vi "Update DVR Constant.vi"() -> ()   [LabVIEW 2020]
uses:
  <vilib>/Utility/traverseref.llb/TRef TravTarget.ctl
  <vilib>/Utility/traverseref.llb/VI Scripting - Traverse.lvlib
panel:
  out "Typedef:Path":path
  out "Class Name":string
  out "VI Name":string
  out "Basic Object Flags":u32
  out "Label.Text":string
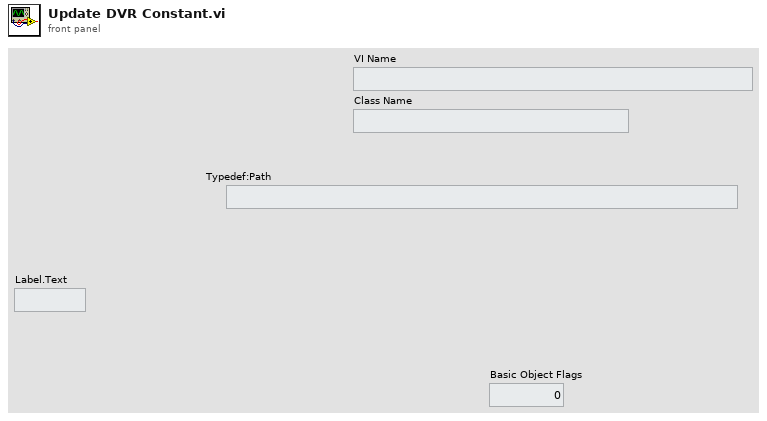
[diagram p1: front panel]
types:
  T1 = typedef "TRef TravTarget.ctl" = enum16{"FP", "BD", "Other"}
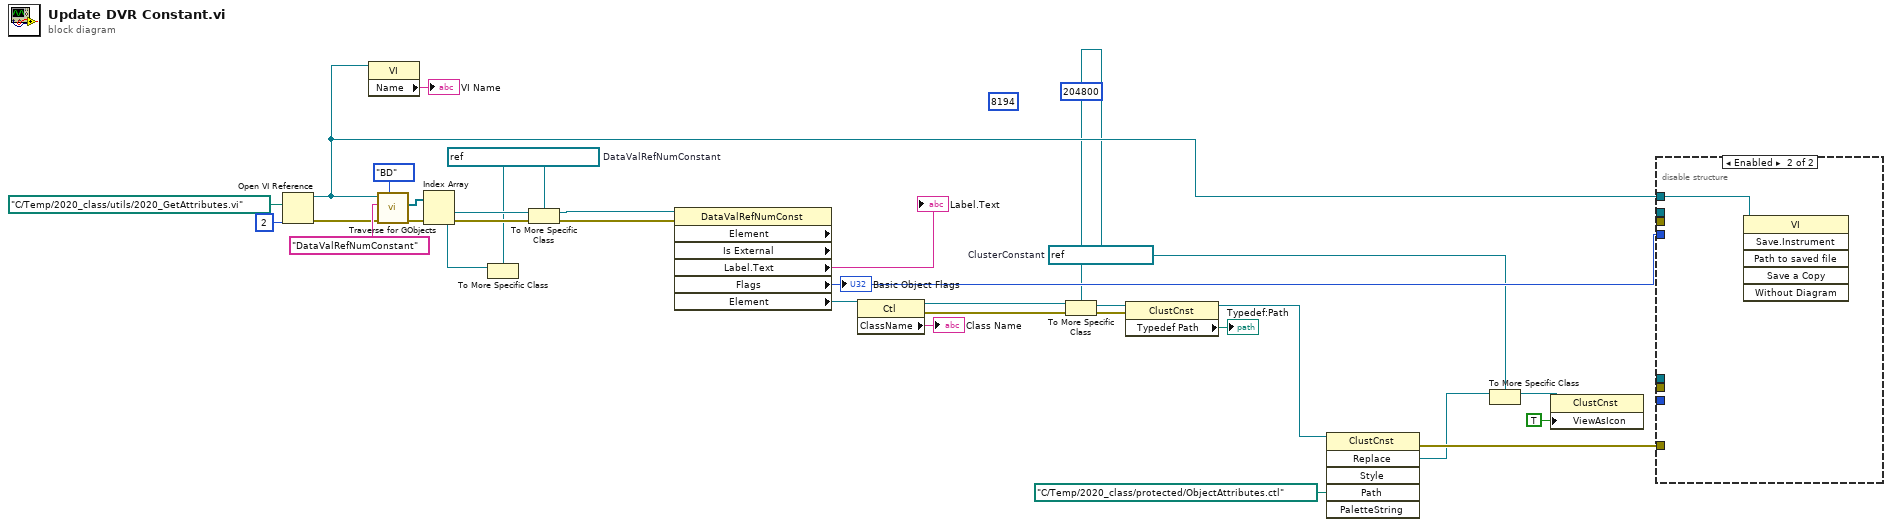
[diagram p0: block diagram]
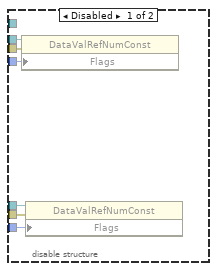
[diagram p2: hidden frame]
diagram:
  w3 = refnum<vi> refnum  # ClusterConstant
  (unwired) u32 204800 ("Basic Object Flags")
  (unwired) u32 8194 ("Basic Object Flags 2")
  w20 = refnum<vi> refnum  # DataValRefNumConstant
  n1 = Open VI Reference(vi path=path "C:/Temp/2020_class/utils/2020_GetAttributes.vi", options=2) -> (vi reference=w15:refnum<vi>, error out=w16:errorcluster)  [unwired: 4 in]
  n2 = property class="VI"(reference=w15) -> ("Name"=→"VI Name":string)  [unwired: 1 in, 2 out]
  n3 = call <vilib>:"Traverse for GObjects.vi"("Traverse Target"=TRef_TravTarget."BD", "error in (no error)"=w16, "Class Name"="DataValRefNumConstant", "VI Refnum"=w15) -> ("error out"=w25:errorcluster, "References"=w27:refnum<vi>[])  [unwired: 4 in, 2 out]
  n4 = Index Array(array=w27) -> (element #1=w26:refnum<vi>, element #2=w21:refnum<vi>)  [unwired: 2 in]
  n5 = To More Specific Class(target class=w20, reference=w21) -> ()  [unwired: 1 in, 2 out]
  n6 = To More Specific Class(target class=w20, reference=w26, error in=w25) -> (specific class reference=w22:refnum<vi>, error out=w24:errorcluster)
  n7 = property class="DataValRefNumConst" props=["Element", "Is External", "Label", "Text", "Flags", "Element"](reference=w22, error in=w24) -> ("Label.Text"=→"Label.Text":string, "Flags"=w19:u32, "Element"=w14:refnum<vi>)  [unwired: 4 out]
  "Basic Object Flags" <- w19
  n8 = property class="Ctl"(reference=w14) -> (reference out=w12:refnum<vi>, error out=w11:errorcluster, "ClassName"=→"Class Name":string)  [unwired: 1 in]
  n9 = To More Specific Class(target class=w3, reference=w12, error in=w11) -> (specific class reference=w9:refnum<vi>, error out=w10:errorcluster)
  n10 = property class="ClustCnst"(reference=w9, error in=w10) -> (reference out=w7:refnum<vi>, "Typedef Path"=→"Typedef:Path":path)  [unwired: 1 out]
  n11 = invoke class="ClustCnst" method="Replace"(reference=w7, "Path"=path "C:/Temp/2020_class/protected/ObjectAttributes.ctl") -> (error out=w5:errorcluster, "Replace"=w4:refnum<vi>)  [unwired: 4 in, 4 out]
  n12 = To More Specific Class(target class=w3, reference=w4) -> (specific class reference=w2:refnum<vi>)  [unwired: 1 in, 1 out]
  n13 = property class="ClustCnst"(reference=w2, "ViewAsIcon"=TRUE ("View As Icon")) -> ()  [unwired: 1 in, 2 out]
  n14 = disable-structure shown="Enabled" {
    disable-tunnel: _ -> [w36 _]
    disable-tunnel: w19 -> [w35 _]
    disable-tunnel: _ -> [w34 _]
    disable-tunnel: _ -> [w33 _]
    disable-tunnel: _ -> [w32 _]
    disable-tunnel: _ -> [w31 _]
    disable-tunnel: w15 -> [_ w37]
    disable-tunnel: w5 -> [_ _]
    frame Disabled {
      n15 = property class="DataValRefNumConst"(reference=w36, error in=w32, "Flags"=w35) -> ()  [unwired: 2 out]
      n16 = property class="DataValRefNumConst"(reference=w34, error in=w31, "Flags"=w33) -> ()  [unwired: 2 out]
    }
    frame Enabled {
      n17 = invoke class="VI" method="Save.Instrument"(reference=w37) -> ()  [unwired: 5 in, 6 out]
    }
  }
